vi "Lab Panel V5.26.vi"() -> ()   [LabVIEW 2017] (continued)
                        n3247 = call "sub vi - temperature delay v3.vi"("2-run"=w5929, "1-run"=w5930, "temp values IN"=w5948, "temp signals"=w5947) -> ("T2-N"=w5942:dbl, "T2-L"=w5943:dbl, "T1-N"=w5944:dbl, "T1-L"=w5945:dbl, "temp values OUT"=w5946:T44)  [unwired: 3 in]
                        n3248 = Unbundle By Name(w5957) -> ("1 (TL) cal"=w5952:dbl, "1 (TN) cal"=w5951:dbl, "2 (TL) cal"=w5950:dbl, "2 (TN) cal"=w5949:dbl)  [unwired: 6 out]
                        n3249 = local write "TEMP LA04"(w5946) -> ()
                        n3250 = Multiply(x=w5945, y=w5952) -> (x*y=w5938:dbl)
                        n3251 = Multiply(x=w5944, y=w5951) -> (x*y=w5937:dbl)
                        n3252 = Multiply(x=w5943, y=w5950) -> (x*y=w5934:dbl)
                        n3253 = Multiply(x=w5942, y=w5949) -> (x*y=w5933:dbl)
                        n3254 = case shown="True" w5929 {
                          tunnel: w5934 -> [w5959 w5964]
                          tunnel: w5939 -> [_ w5962]
                          tunnel: [w5959 w5963] -> w5932
                          tunnel: w5933 -> [w5958 w5961]
                          tunnel: [w5958 w5960] -> w5931
                          frame False {
                          }
                          frame True {
                            n3255 = Multiply(x=w5962, y=w5961) -> (x*y=w5960:dbl)
                            n3256 = Multiply(x=w5962, y=w5964) -> (x*y=w5963:dbl)
                          }
                        }
                        n3257 = case shown="True" w5930 {
                          tunnel: w5938 -> [w5966 w5971]
                          tunnel: w5939 -> [_ w5969]
                          tunnel: [w5966 w5970] -> w5936
                          tunnel: w5937 -> [w5965 w5968]
                          tunnel: [w5965 w5967] -> w5935
                          frame False {
                          }
                          frame True {
                            n3258 = Multiply(x=w5969, y=w5968) -> (x*y=w5967:dbl)
                            n3259 = Multiply(x=w5969, y=w5971) -> (x*y=w5970:dbl)
                          }
                        }
                        n3260 = local read "SIG LAB04-2"() -> (w5954:T2)
                        n3261 = local read "SIG LAB04-1"() -> (w5956:T2)
                        n3262 = Bundle By Name(cluster=w5956, "Tmp Live"=w5936, "Tmp Neut"=w5935) -> (w5955:T2)
                        n3263 = Bundle By Name(cluster=w5954, "Tmp Live"=w5932, "Tmp Neut"=w5931) -> (w5953:T2)
                        n3264 = local write "SIG LAB04-1"(w5955) -> ()
                        n3265 = local write "SIG LAB04-2"(w5953) -> ()
                      }
                      frame #5 {
                        n3266 = case shown="False" w5986 {
                          tunnel: [w6017 w6018] -> w6002
                          tunnel: w5985 -> [_ w6018]
                          frame False {
                            n3267 = local read "CAL LAB05"() -> (w6017:T14)
                          }
                          frame True {
                          }
                        }
                        n3268 = local read "LAB05 TEMP"() -> (w5992:T12)
                        n3269 = local read "TEMP LA05"() -> (w5993:T9)
                        n3270 = call "sub vi - temperature delay v3.vi"("2-run"=w5974, "1-run"=w5975, "temp values IN"=w5993, "temp signals"=w5992) -> ("T2-N"=w5988:dbl, "T2-L"=w5989:dbl, "T1-N"=w5990:dbl, "T1-L"=w5991:dbl, "temp values OUT"=w5987:T44)  [unwired: 3 in]
                        n3271 = local write "TEMP LA05"(w5987) -> ()
                        n3272 = Unbundle By Name(w6002) -> ("1 (TL) cal"=w5994:dbl, "1 (TN) cal"=w5997:dbl, "2 (TL) cal"=w5996:dbl, "2 (TN) cal"=w5995:dbl)  [unwired: 6 out]
                        n3273 = Multiply(x=w5991, y=w5994) -> (x*y=w5983:dbl)
                        n3274 = Multiply(x=w5990, y=w5997) -> (x*y=w5982:dbl)
                        n3275 = Multiply(x=w5989, y=w5996) -> (x*y=w5979:dbl)
                        n3276 = Multiply(x=w5988, y=w5995) -> (x*y=w5978:dbl)
                        n3277 = case shown="True" w5974 {
                          tunnel: w5979 -> [w6004 w6009]
                          tunnel: w5984 -> [_ w6007]
                          tunnel: [w6004 w6008] -> w5977
                          tunnel: w5978 -> [w6003 w6006]
                          tunnel: [w6003 w6005] -> w5976
                          frame False {
                          }
                          frame True {
                            n3278 = Multiply(x=w6007, y=w6006) -> (x*y=w6005:dbl)
                            n3279 = Multiply(x=w6007, y=w6009) -> (x*y=w6008:dbl)
                          }
                        }
                        n3280 = case shown="True" w5975 {
                          tunnel: w5983 -> [w6011 w6016]
                          tunnel: w5984 -> [_ w6014]
                          tunnel: [w6011 w6015] -> w5981
                          tunnel: w5982 -> [w6010 w6013]
                          tunnel: [w6010 w6012] -> w5980
                          frame False {
                          }
                          frame True {
                            n3281 = Multiply(x=w6014, y=w6013) -> (x*y=w6012:dbl)
                            n3282 = Multiply(x=w6014, y=w6016) -> (x*y=w6015:dbl)
                          }
                        }
                        n3283 = local read "SIG LAB05-1"() -> (w6001:T2)
                        n3284 = Bundle By Name(cluster=w6001, "Tmp Live"=w5981, "Tmp Neut"=w5980) -> (w6000:T2)
                        n3285 = local read "SIG LAB05-2"() -> (w5999:T2)
                        n3286 = Bundle By Name(cluster=w5999, "Tmp Live"=w5977, "Tmp Neut"=w5976) -> (w5998:T2)
                        n3287 = local write "SIG LAB05-1"(w6000) -> ()
                        n3288 = local write "SIG LAB05-2"(w5998) -> ()
                      }
                    }
                  }
                }
              }
            }
          }
          frame #22 {
            # "write data to display panel"
            n3289 = global write "Global display 1.vi" "TEST 5-2"(w6053) -> ()
            n3290 = global write "Global display 1.vi" "TEST 4-2"(w6055) -> ()
            n3291 = global write "Global display 1.vi" "TEST 1-2"(w6061) -> ()
            n3292 = global write "Global display 1.vi" "TEST 3-1"(w6058) -> ()
            n3293 = global write "Global display 1.vi" "TEST 5-1"(w6054) -> ()
            n3294 = global write "Global display 1.vi" "TEST 1-1"(w6062) -> ()
            n3295 = global write "Global display 1.vi" "TEST 3-2"(w6057) -> ()
            n3296 = global write "Global display 1.vi" "TEST 4-1"(w6056) -> ()
            n3297 = global write "Global display 1.vi" "TEST 2-2"(w6059) -> ()
            n3298 = global write "Global display 1.vi" "TEST 2-1"(w6060) -> ()
            n3299 = global read "Global display 3.vi" "log 1-1"() -> (→"LOG LAB01-1":string)
            n3300 = global read "Global display 3.vi" "log 3-1"() -> (→"LOG LAB03-1":string)
            n3301 = global read "Global display 3.vi" "log 1-2"() -> (→"LOG LAB01-2":string)
            n3302 = property on="Tab Control 2" class="TabCtl (strict)"() -> ("Pages"=w6052:refnum<vi>[])  [unwired: 2 in, 2 out]
            n3303 = global read "Global display 3.vi" "log 2-1"() -> (→"LOG LAB02-1":string)
            n3304 = global read "Global display 3.vi" "log 2-2"() -> (→"LOG LAB02-2":string)
            n3305 = global read "Global display 3.vi" "log 4-2"() -> (→"LOG LAB04-2":string)
            n3306 = global read "Global display 3.vi" "log 5-2"() -> (→"LOG LAB05-2":string)
            n3307 = global read "Global display 3.vi" "log 5-1"() -> (→"LOG LAB05-1":string)
            n3308 = global read "Global display 3.vi" "log 4-1"() -> (→"LOG LAB04-1":string)
            n3309 = global read "Global display 3.vi" "log 3-2"() -> (→"LOG LAB03-2":string)
            n3310 = Index Array(array=w6052, index=8) -> (element=w6050:refnum<vi>)
            n3311 = property class="Page"(reference=w6050) -> ("PageVis"=w6049:bool)  [unwired: 1 in, 2 out]
            n3312 = global write "Global display 3.vi" "admin"(w6049) -> ()
            n3313 = local read "O/I  LAB05-2"() -> (w6103:bool)
            n3314 = local read "O/I  LAB05-1"() -> (w6104:bool)
            n3315 = local read "O/I  LAB03-2"() -> (w6107:bool)
            n3316 = local read "O/I  LAB04-2"() -> (w6105:bool)
            n3317 = local read "O/I  LAB04-1"() -> (w6106:bool)
            n3318 = local read "O/I  LAB03-1"() -> (w6108:bool)
            n3319 = local read "O/I  LAB01-2"() -> (w6111:bool)
            n3320 = local read "O/I  LAB01-1"() -> (w6112:bool)
            n3321 = local read "O/I  LAB02-1"() -> (w6110:bool)
            n3322 = local read "O/I  LAB02-2"() -> (w6109:bool)
            n3323 = global write "Global display 1.vi" "5-2 O/F"(w6103) -> ()
            n3324 = global write "Global display 1.vi" "5-1 O/F"(w6104) -> ()
            n3325 = global write "Global display 1.vi" "4-1 O/F"(w6106) -> ()
            n3326 = global write "Global display 1.vi" "4-2 O/F"(w6105) -> ()
            n3327 = global write "Global display 1.vi" "3-2 O/F"(w6107) -> ()
            n3328 = global write "Global display 1.vi" "3-1 O/F"(w6108) -> ()
            n3329 = global write "Global display 1.vi" "2-2 O/F"(w6109) -> ()
            n3330 = global write "Global display 1.vi" "2-1 O/F"(w6110) -> ()
            n3331 = global write "Global display 1.vi" "1-2 O/F"(w6111) -> ()
            n3332 = global write "Global display 1.vi" "1-1 O/F"(w6112) -> ()
            n3333 = local read "run lab05-2"() -> (w6093:bool)
            n3334 = local read "run lab04-1"() -> (w6096:bool)
            n3335 = local read "run lab04-2"() -> (w6095:bool)
            n3336 = local read "run lab05-1"() -> (w6094:bool)
            n3337 = local read "TEMP START LAB02-2"() -> (w6035:cluster{"TL":dbl, "TN":dbl})
            n3338 = local read "TEMP START LAB01-2"() -> (w6037:cluster{"TL":dbl, "TN":dbl})
            n3339 = local read "TEMP START LAB02-1"() -> (w6036:cluster{"TL":dbl, "TN":dbl})
            n3340 = local read "TEMP START LAB04-1"() -> (w6032:cluster{"TL":dbl, "TN":dbl})
            n3341 = local read "TEMP START LAB04-2"() -> (w6031:cluster{"TL":dbl, "TN":dbl})
            n3342 = local read "run lab03-2"() -> (w6097:bool)
            n3343 = local read "TEMP START LAB01-1"() -> (w6038:cluster{"TL":dbl, "TN":dbl})
            n3344 = local read "TEMP START LAB05-2"() -> (w6029:cluster{"TL":dbl, "TN":dbl})
            n3345 = local read "TEMP START LAB05-1"() -> (w6030:cluster{"TL":dbl, "TN":dbl})
            n3346 = local read "run lab02-1"() -> (w6100:bool)
            n3347 = local read "run lab03-1"() -> (w6098:bool)
            n3348 = local read "TEMP START LAB03-2"() -> (w6033:cluster{"TL":dbl, "TN":dbl})
            n3349 = local read "run lab01-2"() -> (w6101:bool)
            n3350 = local read "run lab02-2"() -> (w6099:bool)
            n3351 = local read "TEMP START LAB03-1"() -> (w6034:cluster{"TL":dbl, "TN":dbl})
            n3352 = local read "run lab01-1"() -> (w6102:bool)
            n3353 = global write "Global display 1.vi" "5-2 R/S"(w6093) -> ()
            n3354 = global write "Global display 1.vi" "5-1 R/S"(w6094) -> ()
            n3355 = global write "Global display 1.vi" "4-2 R/S"(w6095) -> ()
            n3356 = global write "Global display 1.vi" "4-1 R/S"(w6096) -> ()
            n3357 = global write "Global display 1.vi" "3-2 R/S"(w6097) -> ()
            n3358 = global write "Global display 1.vi" "1-2 R/S"(w6101) -> ()
            n3359 = global write "Global display 1.vi" "2-1 R/S"(w6100) -> ()
            n3360 = global write "Global display 1.vi" "3-1 R/S"(w6098) -> ()
            n3361 = global write "Global display 1.vi" "2-2 R/S"(w6099) -> ()
            n3362 = global write "Global display 1.vi" "1-1 R/S"(w6102) -> ()
            n3363 = global write "Global display 3.vi" "TEMP ST 05-2"(w6029) -> ()
            n3364 = global write "Global display 3.vi" "TEMP ST 05-1"(w6030) -> ()
            n3365 = global write "Global display 3.vi" "TEMP ST 03-2"(w6033) -> ()
            n3366 = global write "Global display 3.vi" "TEMP ST 04-2"(w6031) -> ()
            n3367 = global write "Global display 3.vi" "TEMP ST 01-1"(w6038) -> ()
            n3368 = global write "Global display 3.vi" "TEMP ST 01-2"(w6037) -> ()
            n3369 = global write "Global display 3.vi" "TEMP ST 04-1"(w6032) -> ()
            n3370 = global write "Global display 3.vi" "TEMP ST 02-1"(w6036) -> ()
            n3371 = global write "Global display 3.vi" "TEMP ST 02-2"(w6035) -> ()
            n3372 = global write "Global display 3.vi" "TEMP ST 03-1"(w6034) -> ()
            n3373 = local read "DISP LAB04-2"() -> (w6085:T4)
            n3374 = local read "DISP LAB05-1"() -> (w6084:T4)
            n3375 = local read "DISP LAB04-1"() -> (w6086:T4)
            n3376 = local read "DISP LAB05-2"() -> (w6083:T4)
            n3377 = local read "DISP LAB03-1"() -> (w6088:T4)
            n3378 = local read "DISP LAB03-2"() -> (w6087:T4)
            n3379 = local read "DISP LAB01-2"() -> (w6091:T4)
            n3380 = local read "DISP LAB02-1"() -> (w6090:T4)
            n3381 = local read "DISP LAB02-2"() -> (w6089:T4)
            n3382 = local read "DISP LAB01-1"() -> (w6092:T4)
            n3383 = local read "TEMP RISE LAB05-1"() -> (w6020:cluster{"TL":dbl, "TN":dbl})
            n3384 = local read "TEMP RISE LAB05-2"() -> (w6019:cluster{"TL":dbl, "TN":dbl})
            n3385 = local read "TEMP RISE LAB04-2"() -> (w6021:cluster{"TL":dbl, "TN":dbl})
            n3386 = local read "TEMP RISE LAB04-1"() -> (w6022:cluster{"TL":dbl, "TN":dbl})
            n3387 = local read "TEMP RISE LAB03-2"() -> (w6023:cluster{"TL":dbl, "TN":dbl})
            n3388 = local read "TEMP RISE LAB03-1"() -> (w6024:cluster{"TL":dbl, "TN":dbl})
            n3389 = local read "TEMP RISE LAB01-2"() -> (w6027:cluster{"TL":dbl, "TN":dbl})
            n3390 = local read "TEMP RISE LAB02-2"() -> (w6025:cluster{"TL":dbl, "TN":dbl})
            n3391 = local read "TEMP RISE LAB01-1"() -> (w6028:cluster{"TL":dbl, "TN":dbl})
            n3392 = local read "TEMP RISE LAB02-1"() -> (w6026:cluster{"TL":dbl, "TN":dbl})
            n3393 = global write "Global display 2.vi" "DISP LAB05-1"(w6084) -> ()
            n3394 = global write "Global display 2.vi" "DISP LAB05-2"(w6083) -> ()
            n3395 = global write "Global display 2.vi" "DISP LAB04-2"(w6085) -> ()
            n3396 = global write "Global display 2.vi" "DISP LAB02-1"(w6090) -> ()
            n3397 = global write "Global display 2.vi" "DISP LAB02-2"(w6089) -> ()
            n3398 = global write "Global display 2.vi" "DISP LAB04-1"(w6086) -> ()
            n3399 = global write "Global display 2.vi" "DISP LAB01-2"(w6091) -> ()
            n3400 = global write "Global display 2.vi" "DISP LAB01-1"(w6092) -> ()
            n3401 = global write "Global display 2.vi" "DISP LAB03-1"(w6088) -> ()
            n3402 = global write "Global display 2.vi" "DISP LAB03-2"(w6087) -> ()
            n3403 = global write "Global display 3.vi" "TEMP RS 05-2"(w6019) -> ()
            n3404 = global write "Global display 3.vi" "TEMP RS 05-1"(w6020) -> ()
            n3405 = global write "Global display 3.vi" "TEMP RS 03-2"(w6023) -> ()
            n3406 = global write "Global display 3.vi" "TEMP RS 02-1"(w6026) -> ()
            n3407 = global write "Global display 3.vi" "TEMP RS 02-2"(w6025) -> ()
            n3408 = global write "Global display 3.vi" "TEMP RS 04-2"(w6021) -> ()
            n3409 = global write "Global display 3.vi" "TEMP RS 01-2"(w6027) -> ()
            n3410 = global write "Global display 3.vi" "TEMP RS 03-1"(w6024) -> ()
            n3411 = global write "Global display 3.vi" "TEMP RS 04-1"(w6022) -> ()
            n3412 = global write "Global display 3.vi" "TEMP RS 01-1"(w6028) -> ()
            n3413 = local read "SET LAB05-2"() -> (w6073:T5)
            n3414 = local read "SET LAB05-1"() -> (w6074:T5)
            n3415 = local read "SET LAB04-1"() -> (w6076:T5)
            n3416 = local read "SET LAB04-2"() -> (w6075:T5)
            n3417 = local read "SET LAB03-1"() -> (w6078:T5)
            n3418 = local read "SET LAB03-2"() -> (w6077:T5)
            n3419 = local read "SET LAB02-2"() -> (w6079:T5)
            n3420 = local read "SET LAB01-2"() -> (w6081:T5)
            n3421 = local read "SET LAB02-1"() -> (w6080:T5)
            n3422 = local read "SET LAB01-1"() -> (w6082:T5)
            n3423 = global write "Global display 2.vi" "SET LAB05-2"(w6073) -> ()
            n3424 = global write "Global display 2.vi" "SET LAB05-1"(w6074) -> ()
            n3425 = global write "Global display 2.vi" "SET LAB04-1"(w6076) -> ()
            n3426 = global write "Global display 2.vi" "SET LAB04-2"(w6075) -> ()
            n3427 = global write "Global display 2.vi" "SET LAB03-2"(w6077) -> ()
            n3428 = global write "Global display 2.vi" "SET LAB02-2"(w6079) -> ()
            n3429 = global write "Global display 2.vi" "SET LAB03-1"(w6078) -> ()
            n3430 = global write "Global display 2.vi" "SET LAB01-2"(w6081) -> ()
            n3431 = global write "Global display 2.vi" "SET LAB01-1"(w6082) -> ()
            n3432 = global write "Global display 2.vi" "SET LAB02-1"(w6080) -> ()
            n3433 = local read "RESULT LAB01-1"() -> (w6072:bool)
            n3434 = local read "RESULT LAB03-2"() -> (w6067:bool)
            n3435 = local read "RESULT LAB04-1"() -> (w6066:bool)
            n3436 = local read "RESULT LAB04-2"() -> (w6065:bool)
            n3437 = local read "RESULT LAB02-2"() -> (w6069:bool)
            n3438 = local read "RESULT LAB01-2"() -> (w6071:bool)
            n3439 = local read "RESULT LAB02-1"() -> (w6070:bool)
            n3440 = local read "RESULT LAB03-1"() -> (w6068:bool)
            n3441 = local read "RESULT LAB05-1"() -> (w6064:bool)
            n3442 = local read "RESULT LAB05-2"() -> (w6063:bool)
            n3443 = global write "Global display 2.vi" "RESULT LAB05-1"(w6064) -> ()
            n3444 = global write "Global display 2.vi" "RESULT LAB01-2"(w6071) -> ()
            n3445 = global write "Global display 2.vi" "RESULT LAB03-2"(w6067) -> ()
            n3446 = global write "Global display 2.vi" "RESULT LAB04-1"(w6066) -> ()
            n3447 = global write "Global display 2.vi" "RESULT LAB04-2"(w6065) -> ()
            n3448 = global write "Global display 2.vi" "RESULT LAB05-2"(w6063) -> ()
            n3449 = global write "Global display 2.vi" "RESULT LAB03-1"(w6068) -> ()
            n3450 = global write "Global display 2.vi" "RESULT LAB02-1"(w6070) -> ()
            n3451 = global write "Global display 2.vi" "RESULT LAB02-2"(w6069) -> ()
            n3452 = global write "Global display 2.vi" "RESULT LAB01-1"(w6072) -> ()
          }
          frame #23 {
            # "simulate values"
            n3453 = global write "Global display 4.vi" "LAB deg C"("LAB deg C") -> ()
          }
          frame #24 {
            # "end main and display program"
            n3454 = stacked-sequence {
              seq-local: [_ w6119 _] -> [_ _ w6125]
              tunnel: w6115 -> [w6116 _ _]
              tunnel: w6114 -> [_ _ w6123]
              frame #0 {
                n3455 = case shown="True" w6116 {
                  frame False {
                  }
                  frame True {
                    n3456 = One Button Dialog(message="Excessive number of USB \nresets done, re-start program.") -> ()  [unwired: 1 in, 1 out]
                  }
                }
              }
              frame #1 {
                # "check for reset error"
                n3457 = local read "Simulate"() -> (w6118:bool)
                n3458 = case shown="False" w6118 {
                  tunnel: [w6120 FALSE] -> w6119
                  frame False {
                    n3459 = local read "Reset Error"() -> (w6120:bool)
                    n3460 = case shown="True" w6120 {
                      frame False {
                      }
                      frame True {
                        n3461 = One Button Dialog(message="USB ERROR, program will be stopped.\nClose program, close windows, switch panel off\nand re power panel. If error persists seek help.") -> ()  [unwired: 1 in, 1 out]
                      }
                    }
                  }
                  frame True {
                  }
                }
              }
              frame #2 {
                # "end labview session"
                n3462 = case shown="True" w6123 {
                  frame False {
                  }
                  frame True {
                    n3463 = local read "AI Task2"() -> (w6129:dbl)
                    n3464 = local read "AI Task1"() -> (w6128:dbl)
                    n3465 = local read "AI Task0"() -> (w6127:dbl)
                    n3466 = call "sub vi - AI USB4704 (3)  Close Task v2.vi"(0:w6127, 5:w6128, 7:w6129) -> ()  [unwired: 13 in]
                  }
                }
                n3467 = Or(x=w6125, y="stop all") -> (x .or. y?=w6124:bool)
                n3468 = case shown="True" w6124 {
                  frame False {
                  }
                  frame True {
                    n3469 = stacked-sequence {
                      frame #0 {
                        n3470 = global write "Global display 1.vi" "stop disp"(TRUE) -> ()
                      }
                      frame #1 {
                        n3471 = local read "AI Task2"() -> (w6131:dbl)
                        n3472 = local read "AI Task1"() -> (w6132:dbl)
                        n3473 = local read "AI Task0"() -> (w6133:dbl)
                        n3474 = call "sub vi - AI USB4704 (3)  Close Task v2.vi"(0:w6133, 5:w6132, 7:w6131) -> ()  [unwired: 13 in]
                      }
                      frame #2 {
                        n3475 = Quit LabVIEW(quit? (T)=TRUE) -> ()
                      }
                    }
                  }
                }
              }
            }
          }
        }
        n3476 = node-c288() -> ()  [unwired: 1 in, 1 out]
        "loops" <- w351
      }
      n3477 = node-c288(w323) -> ()  [unwired: 1 out]
    }
  }
